vi "Dual Function.vi"() -> ()   [LabVIEW 2023]
doc: "This example shows that the shapes of dual windows, used for the Gabor transform and expansion, must be close to each other; otherwise, the resulting Gabor coefficients cannot describe the time-varying nature of a signal properly. The shapes of dual windows do not affect perfect reconstruction of the original signal.\n\n<b>Instructions:</b>\n1) Run this VI.\n2) Observe how the design of dual window affects the time-frequency representation of the signal.\n3) Double-click the Dual Window Express VIs on the Block Diagram of this example to understand the settings of the dual windows."
uses:
  Instance           7 21Saved   Dual Function .vi
  <vilib>/addons/Time Frequency Analysis/Transform.llb/TFA Discrete Gabor Transform (Waveform).vi
  <vilib>/addons/Time Frequency Analysis/Transform.llb/TFA Discrete Gabor Expansion (Waveform).vi
  Instance           8 21Saved   Dual Function .vi
  <vilib>/addons/_Advanced Signal Processing/NI_AdvSigProcTFA.lvlib
  <vilib>/Analysis/NI_AALBase.lvlib
panel:
  out "aspt-left-top":bool
  out "Signals_Improper":waveform(dbl)[](graph) caption="Signals"
  out "Signals":waveform(dbl)[](graph)
  out "Magnitude of Gabor Coefficients_Improper":dbl[][](graph) caption="Magnitude of Gabor Coefficients"
  out "Dual Window_Improper":dbl[][](graph) caption="Dual Window"
  out "Dual Window":dbl[][](graph)
  out "Magnitude of Gabor Coefficients":dbl[][](graph)
  # "Overview: Shows that the shapes of dual windows, used for the Gabor transform and expansion, must be close to each other; otherwise, the resulting Gabor coefficients cannot describe the time-varying nature of a signal properly. \nRequirements: LabVIEW Full Development System, Advanced Signal Processing Toolkit\nInstructions: \n1. Run this VI.\n2. Observe how the design of dual window affects the time-frequency representation of the signal.\n3. Double-click the Dual Window Express VIs on the block diagram of this example to understand the settings of the dual windows."
  # "Proper Dual Window"
  # "Improper Dual Window"
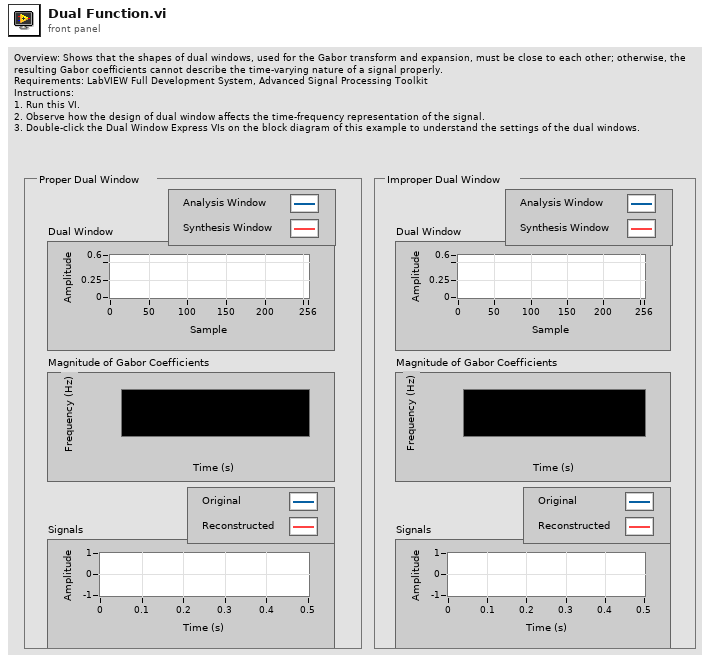
[diagram p1: front panel]
types:
  T1 = cluster{"synthesis window":dbl[], "dM (time steps)":i32, "N (frequency bins)":i32}
  T2 = cluster{"analysis window":dbl[], "dM (time steps)":i32, "N (frequency bins)":i32}
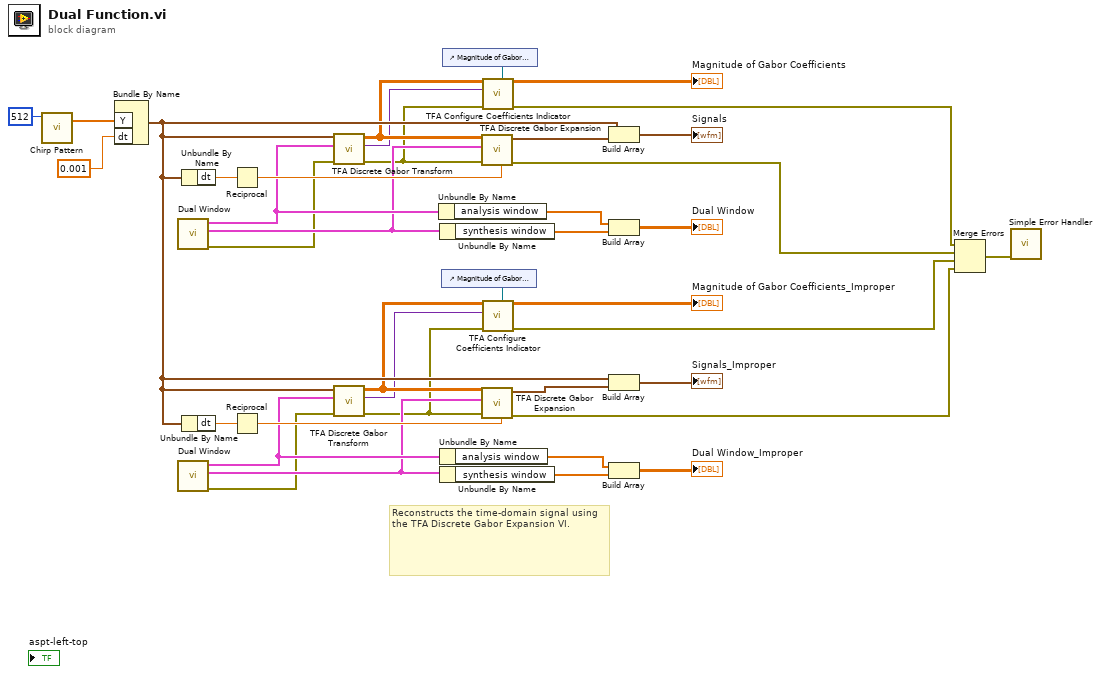
[diagram p0: block diagram]
diagram:
  # "Reconstructs the time-domain signal using the TFA Discrete Gabor Expansion VI."
  n1 = call <vilib>:"Chirp Pattern.vi"("samples"=512) -> ("Chirp Pattern"=w32:dbl[])  [unwired: 3 in, 1 out]
  n2 = Bundle By Name("Y"=w32, "dt"=0.001) -> (w22:waveform(dbl))  [unwired: 1 out]
  n3 = call "Dual Window"() -> ("error out"=w9:errorcluster, "expansion info"=w12:T1, "transform info"=w13:T2)  [unwired: 1 in, 8 out]
  n4 = call "Dual Window"() -> ("error out"=w8:errorcluster, "expansion info"=w10:T1, "transform info"=w11:T2)  [unwired: 1 in, 8 out]
  n5 = Unbundle By Name(w22) -> ("dt"=w26:dbl)
  n6 = Unbundle By Name(w22) -> ("dt"=w24:dbl)
  n7 = Reciprocal(x=w26) -> (1/x=w25:dbl)
  n8 = Reciprocal(x=w24) -> (1/x=w23:dbl)
  n9 = call-poly <vilib>:"TFA Discrete Gabor Transform.vi"("error in (no error)"=w9, "transform info"=w13, "signal"=w22) -> ("error out"=w7:errorcluster, "scale info"=w20:variant, "Gabor coef"=w21:cdb[][])  [unwired: 6 out]
  n10 = call-poly <vilib>:"TFA Discrete Gabor Transform.vi"("error in (no error)"=w8, "transform info"=w11, "signal"=w22) -> ("error out"=w6:errorcluster, "scale info"=w16:variant, "Gabor coef"=w17:cdb[][])  [unwired: 6 out]
  n11 = Unbundle By Name(w13) -> ("analysis window"=w39:dbl[])
  n12 = Unbundle By Name(w12) -> ("synthesis window"=w37:dbl[])
  n13 = Unbundle By Name(w11) -> ("analysis window"=w35:dbl[])
  n14 = Unbundle By Name(w10) -> ("synthesis window"=w36:dbl[])
  n15 = control-ref of="Magnitude of Gabor Coefficients_Improper"() -> (w14:refnum<vi>)
  n16 = control-ref of="Magnitude of Gabor Coefficients"() -> (w18:refnum<vi>)
  n17 = call-poly <vilib>:"TFA Discrete Gabor Expansion.vi"("sampling rate"=w25, "error in (no error)"=w7, "expansion info"=w12, "Gabor coef"=w21) -> ("error out"=w4:errorcluster, "signal"=w30:waveform(dbl))  [unwired: 6 out]
  n18 = call-poly <vilib>:"TFA Discrete Gabor Expansion.vi"("sampling rate"=w23, "error in (no error)"=w6, "expansion info"=w10, "Gabor coef"=w17) -> ("error out"=w3:errorcluster, "signal"=w29:waveform(dbl))  [unwired: 6 out]
  n19 = call <vilib>:"TFA Configure Coefficients Indicator.vi"("reference of TF coefficients indicator"=w18, "error in (no error)"=w7, "scale info"=w20, "TF coefficients"=w21) -> ("error out"=w5:errorcluster, "TF coefficients indicator"=→"Magnitude of Gabor Coefficients":dbl[][])  [unwired: 3 in, 3 out]
  n20 = call <vilib>:"TFA Configure Coefficients Indicator.vi"("reference of TF coefficients indicator"=w14, "error in (no error)"=w6, "scale info"=w16, "TF coefficients"=w17) -> ("error out"=w1:errorcluster, "TF coefficients indicator"=→"Magnitude of Gabor Coefficients_Improper":dbl[][])  [unwired: 3 in, 3 out]
  n21 = Build Array(w22, w30) -> (→"Signals":waveform(dbl)[])
  n22 = Build Array(w39, w37) -> (→"Dual Window":dbl[][])
  n23 = Build Array(w22, w29) -> (→"Signals_Improper":waveform(dbl)[])
  n24 = Build Array(w35, w36) -> (→"Dual Window_Improper":dbl[][])
  n25 = Merge Errors(w5, w4, w1, w3) -> (w2:errorcluster)
  n26 = call <vilib>:"Simple Error Handler.vi"("error in (no error)"=w2) -> ()  [unwired: 4 in, 5 out]
